vi "Download File.vi"(8 "error in (no error)":errorcluster, 9 "File Path":path, 10 "Repository Path":string, 11 "Artifactory in":refnum<class "Artifactory.lvclass">) -> (0 "error out":errorcluster, 1 "File Path out":path, 3 "Artifactory out":refnum<class "Artifactory.lvclass">)   [LabVIEW 2021, in "Artifactory.lvclass"]
uses:
  Artifactory.lvclass
  Actions -- enum.ctl
  Artifactory.lvclass/Artifactory.ctl
  <vilib>/LabVIEW Open Source Project/OpenURI/utilities/Extract URI Components.vi
  <vilib>/Utility/error.llb/Trim Whitespace.vi
  <vilib>/addons/_JKI.lib/REST Client/classes/REST Client/REST Client.lvclass
  <vilib>/addons/_JKI.lib/REST Client/classes/Response Headers/Response Headers.lvclass
  <vilib>/LabVIEW Open Source Project/OpenURI/openURI.lvlib
  <vilib>/httpClient/LabVIEWHTTPClient.lvlib
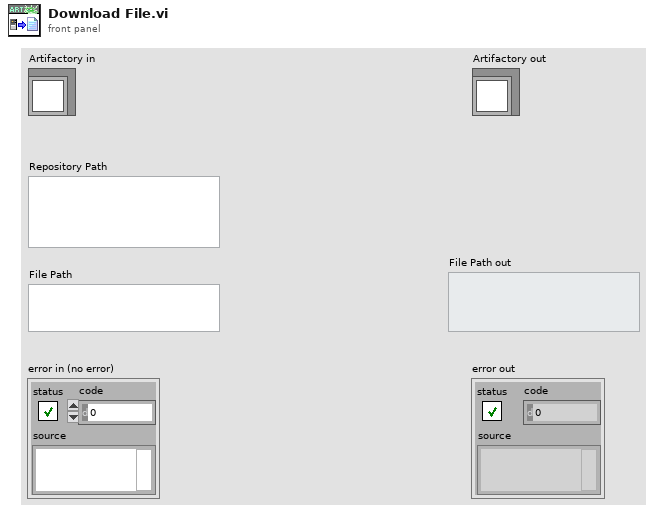
[diagram p1: front panel]
types:
  T1 = typedef "Artifactory.lvclass/Actions -- enum.ctl" = enum16{"Idle", "Custom Event", "Connecting to Artifactory", "Verifying Permissions", "Listing local repository", "Listing remote repository", "Computing changes", "Uploading file", "Downloading file"}
  T2 = typedef "LabVIEWHTTPClient.lvlib/ClientHandle.ctl" = refnum<k1>
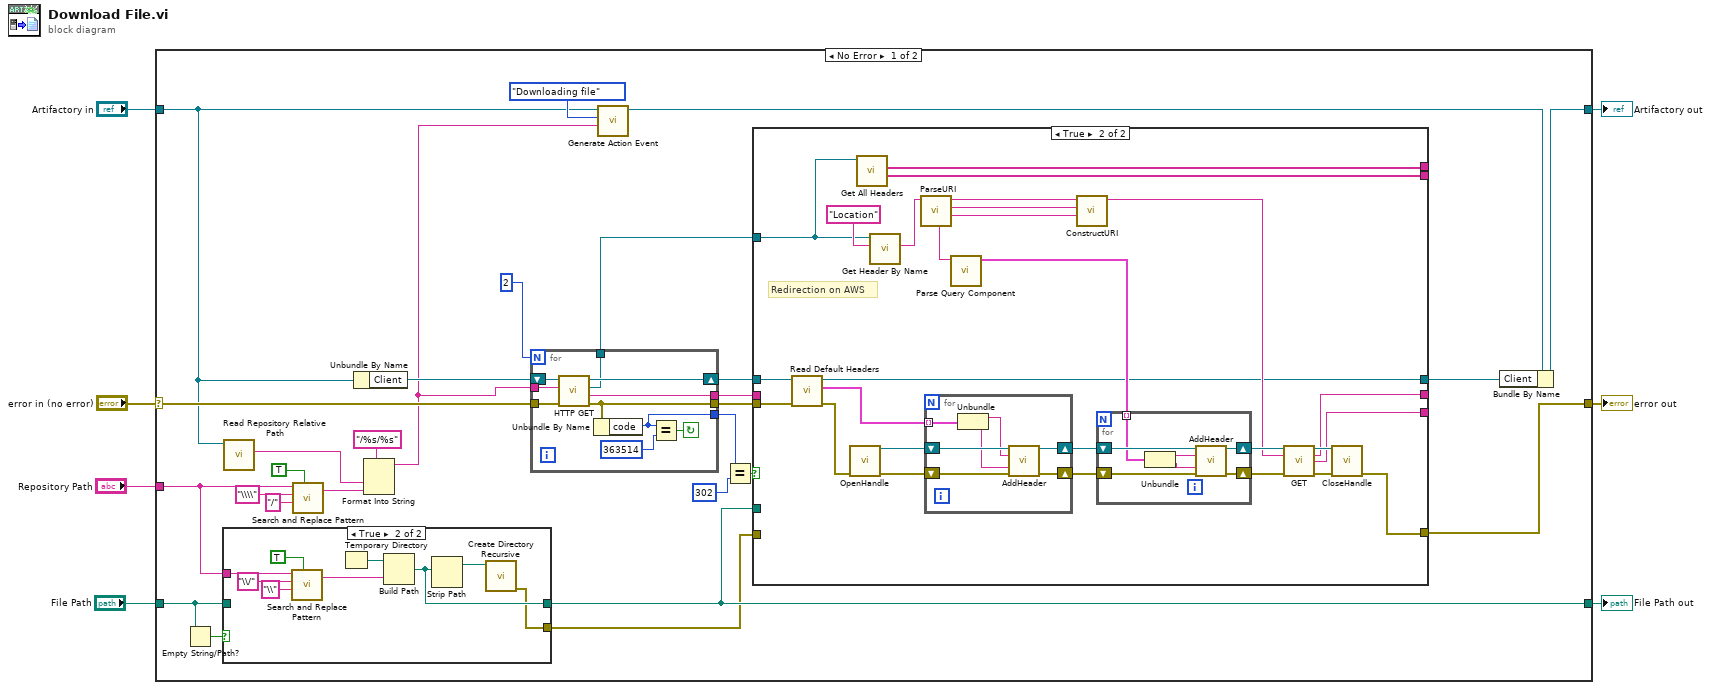
[diagram p0: block diagram]
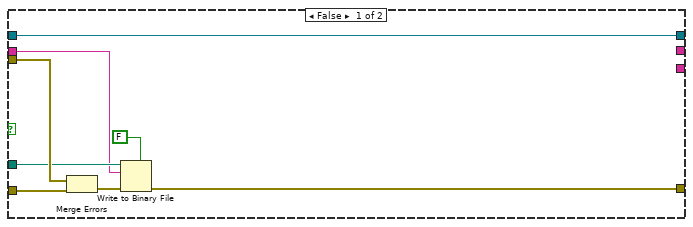
[diagram p2: hidden frame]
diagram:
  n1 = case shown="No Error" "error in (no error)" {
    selector: "error in (no error)" -> [w29 w106]
    tunnel: [w8 w106] -> w6
    tunnel: [w28 w105] -> w4
    tunnel: "Artifactory in" -> [w21 w105]
    tunnel: "Repository Path" -> [w24 _]
    tunnel: "File Path" -> [w25 _]
    tunnel: [w10 _] -> w1
    frame No Error {
      n2 = Empty String/Path?(string/path=w25) -> (empty?=w26:bool)
      n3 = case shown="True" w26 {
        tunnel: w24 -> [_ w99]
        tunnel: w25 -> [w95 _]
        tunnel: [w95 w97] -> w10
        tunnel: [_ w96] -> w9
        frame False {
        }
        frame True {
          n4 = call <vilib>:"Search and Replace Pattern.vi"("string"=w99, "regular expression (\"\")"="\\/" ("regular expression (\"\")"), "replace string (\"\")"="\\" ("regular expression (\"\")"), "replace all? (F)"=TRUE) -> ("result string"=w100:string)  [unwired: 1 in, 1 out]
          n5 = Temporary Directory() -> (w104:path)
          n6 = Build Path(base path=w104, name or relative path=w100) -> (appended path=w97:path)
          n7 = Strip Path(path=w97) -> (stripped path=w98:path)  [unwired: 1 out]
          n8 = call <vilib>:"Create Directory Recursive.vi"("directory"=w98) -> ("error out"=w96:errorcluster)  [unwired: 4 in, 2 out]
        }
      }
      n9 = call "Read Repository Relative Path.vi"("Artifactory in"=w21) -> ("repository path"=w27:string)  [unwired: 9 in, 1 out]
      n10 = call <vilib>:"Search and Replace Pattern.vi"("string"=w24, "regular expression (\"\")"="\\\\" ("regular expression (\"\")"), "replace string (\"\")"="/" ("regular expression (\"\")"), "replace all? (F)"=TRUE) -> ("result string"=w30:string)  [unwired: 1 in, 1 out]
      n11 = Unbundle By Name(w21) -> ("Client"=w34:refnum<class "REST Client.lvclass">)
      n12 = Format Into String(format string="/%s/%s" ("Path"), w27, w30) -> (resulting string=w20:string)  [unwired: 2 in, 1 out]
      n13 = for {
        N: 2 -> [_]
        tunnel: w20 -> [w93]
        shift-right: [w91] -> w15
        shift-left: w34 -> [w94]
        tunnel: w29 -> [w92]
        tunnel: [w90] -> w12
        tunnel: [w87] -> w13
        tunnel: [w86] -> w11
        tunnel: [w85] -> w17
        stop <- w88 continue-if-true
        n14 = call-dynamic "HTTP GET.vi"("error in (no error)"=w92, "Path"=w93, "REST Client in"=w94) -> ("error out"=w90:errorcluster, "Response body"=w87:string, "Response Headers"=w86:refnum<class "Response Headers.lvclass">, "REST Client out"=w91:refnum<class "REST Client.lvclass">)  [unwired: 3 in, 2 out]
        n15 = Unbundle By Name(w90) -> ("code"=w85:i32)
        n16 = Equal?(x=w85, y=363514) -> (x = y?=w88:bool)
      }
      n17 = call-dynamic "Generate Action Event.vi"("Description"=w20, "Action"=Actions_--_enum."Downloading file", "Artifactory in"=w21) -> ("Artifactory out"=w22:refnum<class "Artifactory.lvclass">)  [unwired: 7 in, 1 out]
      n18 = Equal?(x=w17, y=302) -> (x = y?=w16:bool)
      n19 = case shown="True" w16 {
        tunnel: w15 -> [w43 w49]
        tunnel: [w43 w50] -> w14
        tunnel: w13 -> [w37 _]
        tunnel: w12 -> [w39 w47]
        tunnel: w11 -> [_ w56]
        tunnel: [_ w69] -> _
        tunnel: [_ w68] -> _
        tunnel: w10 -> [w38 _]
        tunnel: w9 -> [w40 _]
        tunnel: [w36 w51] -> w8
        tunnel: [_ w45] -> _
        tunnel: [_ w44] -> _
        frame False {
          n20 = Merge Errors(w39, w40) -> (w42:errorcluster)
          n21 = Write to Binary File(file (use dialog)=w38, data=w37, error in=w42, 5:FALSE ("prepend array or string size? (T)")) -> (error out=w36:errorcluster)  [unwired: 2 in, 2 out]
        }
        frame True {
          # "Redirection on AWS"
          n22 = call-dynamic "Read Default Headers.vi"("error in (no error)"=w47, "REST Client in"=w49) -> ("error out"=w48:errorcluster, "Headers"=w46:cluster{"header":string, "value":string}[], "REST Client out"=w50:refnum<class "REST Client.lvclass">)  [unwired: 7 in]
          n23 = call <vilib>:"OpenHandle.vi"("error in (no error)"=w48) -> ("client handle out"=w53:T2, "error out"=w55:errorcluster)  [unwired: 13 in]
          n24 = call <vilib>:"Get All Headers.vi"("Response Headers in"=w56) -> ("Values"=w68:string[], "Names"=w69:string[])  [unwired: 7 in, 2 out]
          n25 = call <vilib>:"Get Header By Name.vi"("Name"="Location" ("Path"), "Response Headers in"=w56) -> ("Value"=w63:string)  [unwired: 6 in, 3 out]
          n26 = call <vilib>:"ParseURI.vi"("URI"=w63) -> ("path"=w65:string, "authority"=w66:string, "scheme"=w67:string, "query"=w64:string)  [unwired: 5 in, 2 out]
          n27 = for {
            shift-right: [w76] -> w54
            shift-left: w55 -> [w77]
            shift-right: [w74] -> w52
            shift-left: w53 -> [w75]
            tunnel: w46 -> [w73] mode=indexing
            n28 = Unbundle(w73) -> ("header"=w72:string, "value"=w71:string)
            n29 = call <vilib>:"AddHeader.vi"("client handle"=w75, "header"=w72, "value"=w71, "error in (no error)"=w77) -> ("client handle out"=w74:T2, "error out"=w76:errorcluster)  [unwired: 10 in]
          }
          n30 = call <vilib>:"Parse Query Component.vi"("query"=w64) -> ("Query"=w57:cluster{"argument":string, "value":string}[])  [unwired: 10 in]
          n31 = call <vilib>:"ConstructURI.vi"("path component"=w65, "authority"=w66, "scheme"=w67) -> ("URI"=w58:string)  [unwired: 7 in, 1 out]
          n32 = for {
            shift-right: [w84] -> w62
            shift-left: w52 -> [w82]
            shift-right: [w83] -> w61
            shift-left: w54 -> [w81]
            tunnel: w57 -> [w80] mode=indexing
            n33 = Unbundle(w80) -> ("argument"=w79:string, "value"=w78:string)
            n34 = call <vilib>:"AddHeader.vi"("client handle"=w82, "header"=w79, "value"=w78, "error in (no error)"=w81) -> ("client handle out"=w84:T2, "error out"=w83:errorcluster)  [unwired: 10 in]
          }
          n35 = call <vilib>:"GET.vi"("client handle"=w62, "url"=w58, "error in (no error)"=w61) -> ("client handle out"=w60:T2, "headers"=w44:string, "body"=w45:string, "error out"=w59:errorcluster)  [unwired: 9 in]
          n36 = call <vilib>:"CloseHandle.vi"("client handle"=w60, "error in (no error)"=w59) -> ("error out"=w51:errorcluster)  [unwired: 13 in]
        }
      }
      n37 = Bundle By Name(cluster=w22, "Client"=w14) -> (w28:refnum<class "Artifactory.lvclass">)
    }
    frame Error {
    }
  }
  "error out" <- w6
  "Artifactory out" <- w4
  "File Path out" <- w1
